vi "Block Read Raw To Scaled Value.vi"(1 "Scaling Constants":T1, 2 "u16 Raw Value":u16[](array[numeric])) -> (7 "dbl Scaled Value":dbl[](array[numeric]))   [LabVIEW 2021]
uses:
  <vilib>/myRIO/Common/Instrument Driver Framework/Utilities/typedefs/Analog Scaling Constants.ctl
panel:
  # "Converts raw ADC u16 values to scaled dbl values based on the scaling constants."
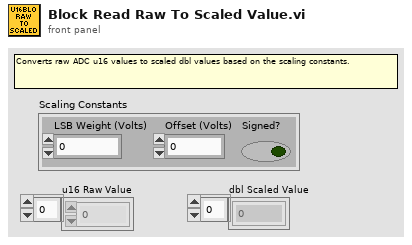
[diagram p1: front panel]
types:
  T1 = typedef "Analog Scaling Constants.ctl" = cluster{"LSB Weight (Volts)":dbl, "Offset (Volts)":dbl, "Signed?":bool}
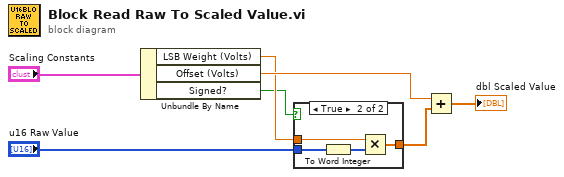
[diagram p0: block diagram]
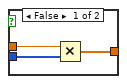
[diagram p2: hidden frame]
diagram:
  n1 = Unbundle By Name("Scaling Constants") -> ("LSB Weight (Volts)"=w3:dbl, "Offset (Volts)"=w6:dbl, "Signed?"=w2:bool)
  n2 = case shown="True" w2 {
    tunnel: "u16 Raw Value" -> [w10 w13]
    tunnel: w3 -> [w9 w12]
    tunnel: [w8 w11] -> w1
    frame False {
      n3 = Multiply(x=w9, y=w10) -> (x*y=w8:dbl[])
    }
    frame True {
      n4 = To Word Integer(number=w13) -> (16bit integer=w14:i16[])
      n5 = Multiply(x=w12, y=w14) -> (x*y=w11:dbl[])
    }
  }
  n6 = Add(x=w6, y=w1) -> (x+y=→"dbl Scaled Value":dbl[])
